vi "stop.vi"(8 "error in (no error)":errorcluster, 11 "ScanHeadAK130114ResonanceFlexRIO in":refnum<class "ScanHeadAK130114ResonanceFlexRIO.lvclass">) -> (0 "error out":errorcluster, 3 "ScanHeadAK130114ResonanceFlexRIO out":refnum<class "ScanHeadAK130114ResonanceFlexRIO.lvclass">)   [LabVIEW 2010, in "ScanHeadAK130114ResonanceFlexRIO.lvclass"]
uses:
  ScanHeadAK130114ResonanceFlexRIO.lvclass
  Trajectory/GenericTrajectory/GenericTrajectory/GenericTrajectory.lvclass
  Trajectory/TrajectoryMG100122GenericFPGA/TrajectoryMG100122GenericFPGA/TrajectoryMG100122GenericFPGA.lvclass
  common/classes/ErrorController/ErrorController/class_data.vi
  common/classes/ErrorController/ErrorController/ErrorController.lvclass
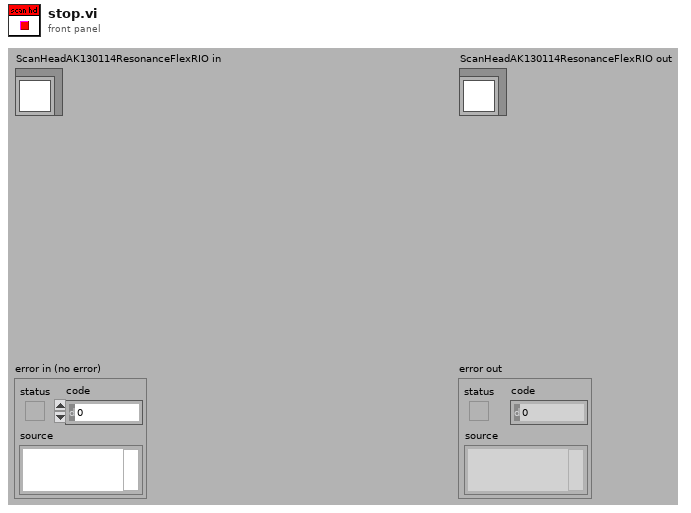
[diagram p1: front panel]
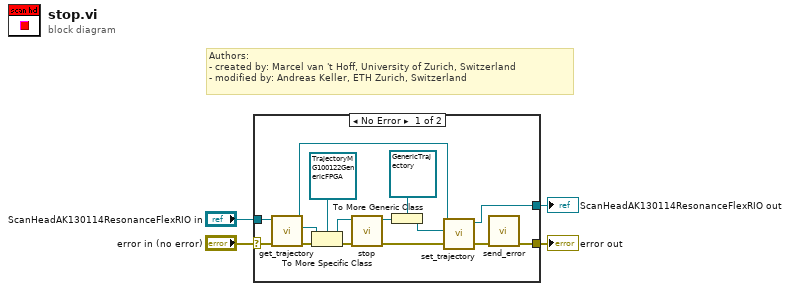
[diagram p0: block diagram]
diagram:
  # "Authors: \n- created by: Marcel van 't Hoff, University of Zurich, Switzerland\n- modified by: Andreas Keller, ETH Zurich, Switzerland"
  n1 = case shown="No Error" "error in (no error)" {
    selector: "error in (no error)" -> [w14 w20]
    tunnel: [w6 w20] -> w3
    tunnel: [w5 w21] -> w2
    tunnel: "ScanHeadAK130114ResonanceFlexRIO in" -> [w9 w21]
    frame No Error {
      n2 = call-dynamic "get_trajectory.vi"("error in (no error)"=w14, "GenericScanHead.lvclass in"=w9) -> ("error out"=w19:errorcluster, "trajectory"=w18:refnum<class "GenericTrajectory.lvclass">, "GenericScanHead.lvclass out"=w10:refnum<class "ScanHeadAK130114ResonanceFlexRIO.lvclass">)  [unwired: 7 in]
      n3 = To More Specific Class(target class=refnum<class "TrajectoryMG100122GenericFPGA.lvclass"> refnum ("TrajectoryMG100122GenericFPGA.lvclass"), reference=w18, error in=w19) -> (specific class reference=w8:refnum<class "TrajectoryMG100122GenericFPGA.lvclass">, error out=w16:errorcluster)
      n4 = call-dynamic "stop.vi"("error in (no error)"=w16, "TrajectoryMG100122GenericFPGA in"=w8) -> ("error out"=w15:errorcluster, "TrajectoryMG100122GenericFPGA out"=w13:refnum<class "TrajectoryMG100122GenericFPGA.lvclass">)  [unwired: 8 in]
      n5 = To More Generic Class(target class=refnum<class "GenericTrajectory.lvclass"> refnum ("GenericTrajectory.lvclass"), reference=w13) -> (generic class reference=w11:refnum<class "GenericTrajectory.lvclass">)
      n6 = call-dynamic "set_trajectory.vi"("error in (no error)"=w15, "trajectory"=w11, "GenericScanHead.lvclass in"=w10) -> ("error out"=w7:errorcluster, "GenericScanHead.lvclass out"=w5:refnum<class "ScanHeadAK130114ResonanceFlexRIO.lvclass">)  [unwired: 7 in]
      n7 = call "send_error.vi"("error in (no error)"=w7) -> ("error out"=w6:errorcluster)  [unwired: 10 in]
    }
    frame Error {
    }
  }
  "error out" <- w3
  "ScanHeadAK130114ResonanceFlexRIO out" <- w2
